vi "RTLSDR Open And Set Defaults.vi"(8 "error in (no error)":errorcluster) -> (0 "error out":errorcluster)   [LabVIEW 2017]
doc: "Opens the RTL-SDR device and sets default acquisition parameters."
uses:
  RTLSDR Global Variables.vi
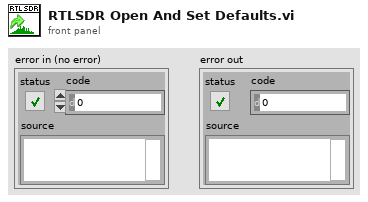
[diagram p1: front panel]
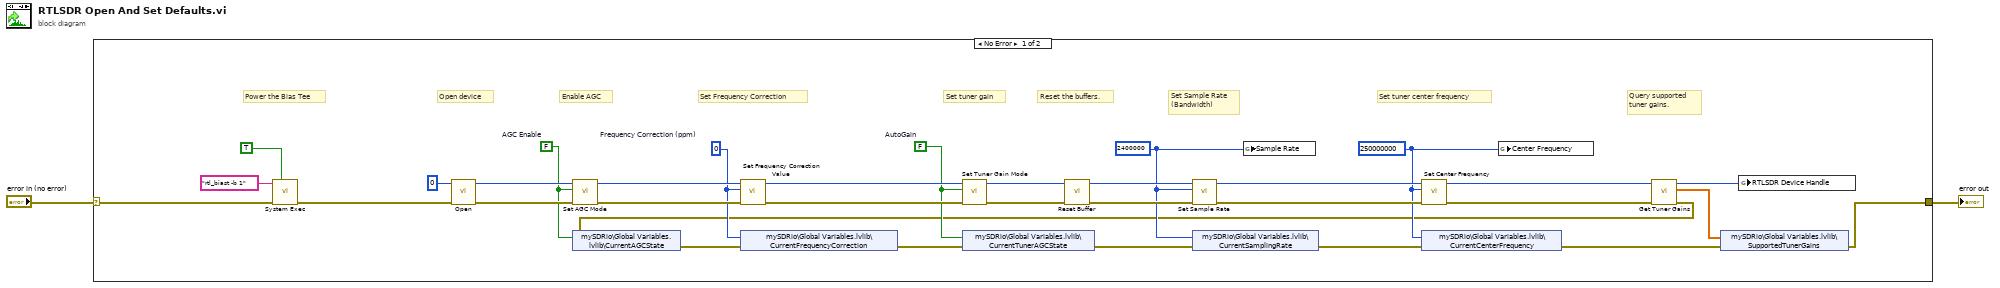
[diagram p0: block diagram]
diagram:
  n1 = case shown="No Error" "error in (no error)" {
    selector: "error in (no error)" -> [w5 w36]
    tunnel: [w7 w36] -> w2
    frame No Error {
      w14 = u32 250000000 ("Center Frequency")
      w17 = u32 2400000 ("Sample Rate")
      w20 = FALSE  # AutoGain
      w21 = 0  # Frequency Correction (ppm)
      w22 = FALSE  # AGC Enable
      # "Power the Bias Tee"
      # "Query supported\ntuner gains."
      # "Set tuner center frequency"
      # "Set Sample Rate\n(Bandwidth)"
      # "Reset the buffers."
      # "Set tuner gain"
      # "Set Frequency Correction"
      # "Enable AGC"
      # "Open device"
      n2 = call <vilib>:"System Exec.vi"("wait until completion? (T)"=TRUE, "error in (no error)"=w5, "command line"="rtl_biast -b 1") -> ("error out"=w6:errorcluster)  [unwired: 5 in, 3 out]
      n3 = call "Open.vi"("error in (no error)"=w6, "Device Index"=u32 0) -> ("error out"=w24:errorcluster, "DeviceRefnum Out"=w25:u64)  [unwired: 6 in]
      n4 = call "Set AGC Mode.vi"("error in (no error)"=w24, "AGC Enable"=w22, "DeviceRefnum"=w25) -> ("error out"=w26:errorcluster, "DeviceRefnum Out"=w27:u64)  [unwired: 6 in, 1 out]
      n5 = call "Set Frequency Correction Value.vi"("error in (no error)"=w26, "Frequency Correction (ppm)"=w21, "DeviceRefnum"=w27) -> ("error out"=w28:errorcluster, "DeviceRefnum Out"=w29:u64)  [unwired: 6 in, 1 out]
      n6 = call "Set Tuner Gain Mode.vi"("error in (no error)"=w28, "AutoGain"=w20, "DeviceRefnum"=w29) -> ("error out"=w30:errorcluster, "DeviceRefnum Out"=w31:u64)  [unwired: 6 in, 1 out]
      n7 = call "Reset Buffer.vi"("error in (no error)"=w30, "DeviceRefnum"=w31) -> ("error out"=w32:errorcluster, "DeviceRefnum Out"=w33:u64)  [unwired: 7 in, 1 out]
      n8 = call "Set Sample Rate.vi"("error in (no error)"=w32, "Sample Rate"=w17, "DeviceRefnum"=w33) -> ("error out"=w34:errorcluster, "DeviceRefnum Out"=w35:u64)  [unwired: 6 in, 1 out]
      n9 = global write "RTLSDR Global Variables.vi" "Sample Rate"(w17) -> ()
      n10 = call "Set Center Frequency.vi"("error in (no error)"=w34, "Center Frequency"=w14, "DeviceRefnum"=w35) -> ("error out"=w11:errorcluster, "DeviceRefnum Out"=w13:u64)  [unwired: 6 in, 1 out]
      n11 = global write "RTLSDR Global Variables.vi" "Center Frequency"(w14) -> ()
      n12 = call "Get Tuner Gains.vi"("error in (no error)"=w11, "DeviceRefnum"=w13) -> ("error out"=w10:errorcluster, "Supported Gains"=w8:dbl[], "DeviceRefnum Out"=w12:u64)  [unwired: 7 in]
      n13 = shared-variable "mySDRio\\Global Variables.lvlib\\CurrentAGCState"(w22, error in=w10) -> (error out=w19:errorcluster)
      n14 = shared-variable "mySDRio\\Global Variables.lvlib\\CurrentFrequencyCorrection"(w21, error in=w19) -> (error out=w18:errorcluster)
      n15 = shared-variable "mySDRio\\Global Variables.lvlib\\CurrentTunerAGCState"(w20, error in=w18) -> (error out=w16:errorcluster)
      n16 = shared-variable "mySDRio\\Global Variables.lvlib\\CurrentSamplingRate"(w17, error in=w16) -> (error out=w15:errorcluster)
      n17 = shared-variable "mySDRio\\Global Variables.lvlib\\CurrentCenterFrequency"(w14, error in=w15) -> (error out=w9:errorcluster)
      n18 = shared-variable "mySDRio\\Global Variables.lvlib\\SupportedTunerGains"(w8, error in=w9) -> (error out=w7:errorcluster)
      n19 = global write "RTLSDR Global Variables.vi" "RTLSDR Device Handle"(w12) -> ()
    }
    frame Error {
    }
  }
  "error out" <- w2
